vi "Pattern_mover_v1.vi"() -> ()   [LabVIEW 2014]
uses:
  <userlib>/Nanonis Prog Interface V5/Nanonis Prog Interface.lvlib
panel:
  in  "y":sgl format="%#_6p"
  in  "x":sgl format="%#_6p"
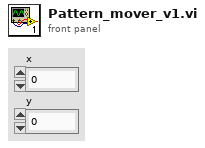
[diagram p1: front panel]
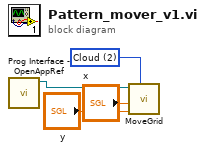
[diagram p0: block diagram]
diagram:
  w3 = u16 2 items=["Line", "Grid", "Cloud"] ("type")
  n1 = call <userlib>:"Prog Interface - OpenAppRef.vi"() -> ("Application reference"=w4:refnum<vi>)  [unwired: 6 in, 1 out]
  n2 = call "MoveGrid.vi"("type"=w3, "y"="y", "x"="x", "Application ref in"=w4) -> ()  [unwired: 6 in, 2 out]
